vi "SDSU_SetInitVals.vi"(0 "ConfigPath":path, 11 "error in":errorcluster) -> (6 "supabort":bool, 8 "libdir out":path, 10 "cmdtrans out":path, 15 "error out":errorcluster)   [LabVIEW 2016]
uses:
  DHE/private/vis/DHE_Device.ctl
  SDSU_GBLVariables.vi
  DBSHAND/private/vis/DatabaseHand_Element_Set(string).vi
panel:
  in  "supinttime":bool
  in  "cmdtrans":path=path ""
  in  "devparams":string
  in  "libdir":path=path ""
  in  "linktype":string="genIII"
  in  "devtype":string="pcix"
  in  "mapsize":i32=-1
  in  "exp_overhead":string
  in  "minexptime":string
  in  "seq_overhead":string
  in  "Device In":T1 {"readtime" format="%.2f"}
  in  "suphardtime":bool
  in  "devno":i32
  in  "supabortctrl":bool
  in  "overhead":sgl=-1.0 format="%.2f"
  in  "ShiftedPix":i32=-1
  in  "bpp":i32=16
  in  "modifiers":string
  in  "FPA":string
  in  "readoutmode":string
  in  "ConfigVariables":string[][](table)=[["Device", "devno", "SDSU_SetInitVals.vi", "devno", "0", "I32"], ["Device", "mapsize", "SDSU_SetInitVals.vi", "mapsize", "", "I32"], ["Device", "params", "SDSU_SetInitVals.vi", "devparams", "", "STR"], ["Device", "type", "SDSU_SetInitVals.vi", "devtype", "", "STR"], ["Device", "link", "SDSU_SetInitVals.vi", "linktype", "", "STR"], ["Device", "libdir", "SDSU_SetInitVals.vi", "libdir", "", "Path"], ["Lod", "Utility", "SDSU_SetInitVals.vi", "Utility Path", "none", "Path"], ["Lod", "Timing", "SDSU_SetInitVals.vi", "Timing Path", "none", "Path"], ["Lod", "Pci", "SDSU_SetInitVals.vi", "Pci Path", "none", "Path"], ["Geometry", "FPA", "SDSU_SetInitVals.vi", "FPA", "", "STR"], ["Geometry", "modifiers", "SDSU_SetInitVals.vi", "modifiers", "", "STR"], ["FPA", "name", "SDSU_SetInitVals.vi", "FPA", "", "STR"], ["FPA", "modifiers", "SDSU_SetInitVals.vi", "modifiers", "", "STR"], ["FPA", "readmode", "SDSU_SetInitVals.vi", "readoutmode", "", "STR"], ["Roi", "Xstart", "SDSU_SetInitVals.vi", "xstart", "1", "U32"], ["Roi", "Xsize", "SDSU_SetInitVals.vi", "xsize", "2048", "U32"], ["Roi", "Ystart", "SDSU_SetInitVals.vi", "ystart", "1", "U32"], ["Roi", "Ysize", "SDSU_SetInitVals.vi", "ysize", "2048", "U32"], ["Binning", "X", "SDSU_SetInitVals.vi", "xbin", "1", "U32"], ["Binning", "Y", "SDSU_SetInitVals.vi", "ybin", "1", "U32"], ["Misc", "ReadoutMode", "SDSU_SetInitVals.vi", "readoutmode", "left", "STR"], ["Misc", "Temperature", "SDSU_SetInitVals.vi", "CCDTemperature", "-110", "I32"], ["Misc", "Commands", "SDSU_SetInitVals.vi", "CommandStr", "", "STR"], ["Misc", "bpp", "SDSU_SetInitVals.vi", "bpp", "16", "I32"], ["Misc", "min_exptime", "SDSU_SetInitVals.vi", "min_exptime", "0", "SGL"], ["Misc", "transfile", "SDSU_SetInitVals.vi", "cmdtrans", "", "PATH"], ["Readout", "PixelTime", "SDSU_SetInitVals.vi", "PixelTime", "3", "SGL"], ["Readout", "SkipPixel", "SDSU_SetInitVals.vi", "SkipPixel", "0", "SGL"], ["Readout", "SkipRow", "SDSU_SetInitVals.vi", "SkipRow", "0", "SGL"], ["Readout", "ShiftRow", "SDSU_SetInitVals.vi", "ShiftRow", "0", "SGL"], ["Readout", "ShiftedPix", "SDSU_SetInitVals.vi", "ShiftedPix", "0", "I32"], ["Readout", "known_overhead", "SDSU_SetInitVals.vi", "overhead", "0", "SGL"], ["Readout", "frame_overhead", "SDSU_SetInitVals.vi", "overhead", "0", "SGL"], ["Readout", "seq_overhead", "SDSU_SetInitVals.vi", "seq_overhead", "0", "STR"], ["Readout", "exp_overhead", "SDSU_SetInitVals.vi", "exp_overhead", "0", "STR"], ["Readout", "minexptime", "SDSU_SetInitVals.vi", "minexptime", "0", "STR"], ["Readout", "support_abort", "SDSU_SetInitVals.vi", "supabortctrl", "", "BOOL"], ["Readout", "support_hardtime", "SDSU_SetInitVals.vi", "suphardtime", "", "BOOL"], ["Readout", "support_actual_inttime", "SDSU_SetInitVals.vi", "supinttime", "", "BOOL"]]
  in  "Pci Path":path=path "none"
  in  "ShiftRow":sgl=-1.0 format="%.2f"
  in  "SkipRow":sgl=-1.0 format="%.2f"
  in  "SkipPixel":sgl=-1.0 format="%.2f"
  in  "PixelTime":sgl=-1.0 format="%.2f"
  in  "CommandStr":string
  in  "min_exptime":sgl
  in  "Commnds To Execute after set":i32(listbox)
  in  "Timing Path":path=path "none"
  in  "Utility Path":path=path "none"
  in  "CCDTemperature":i32=-110
  # "Misc"
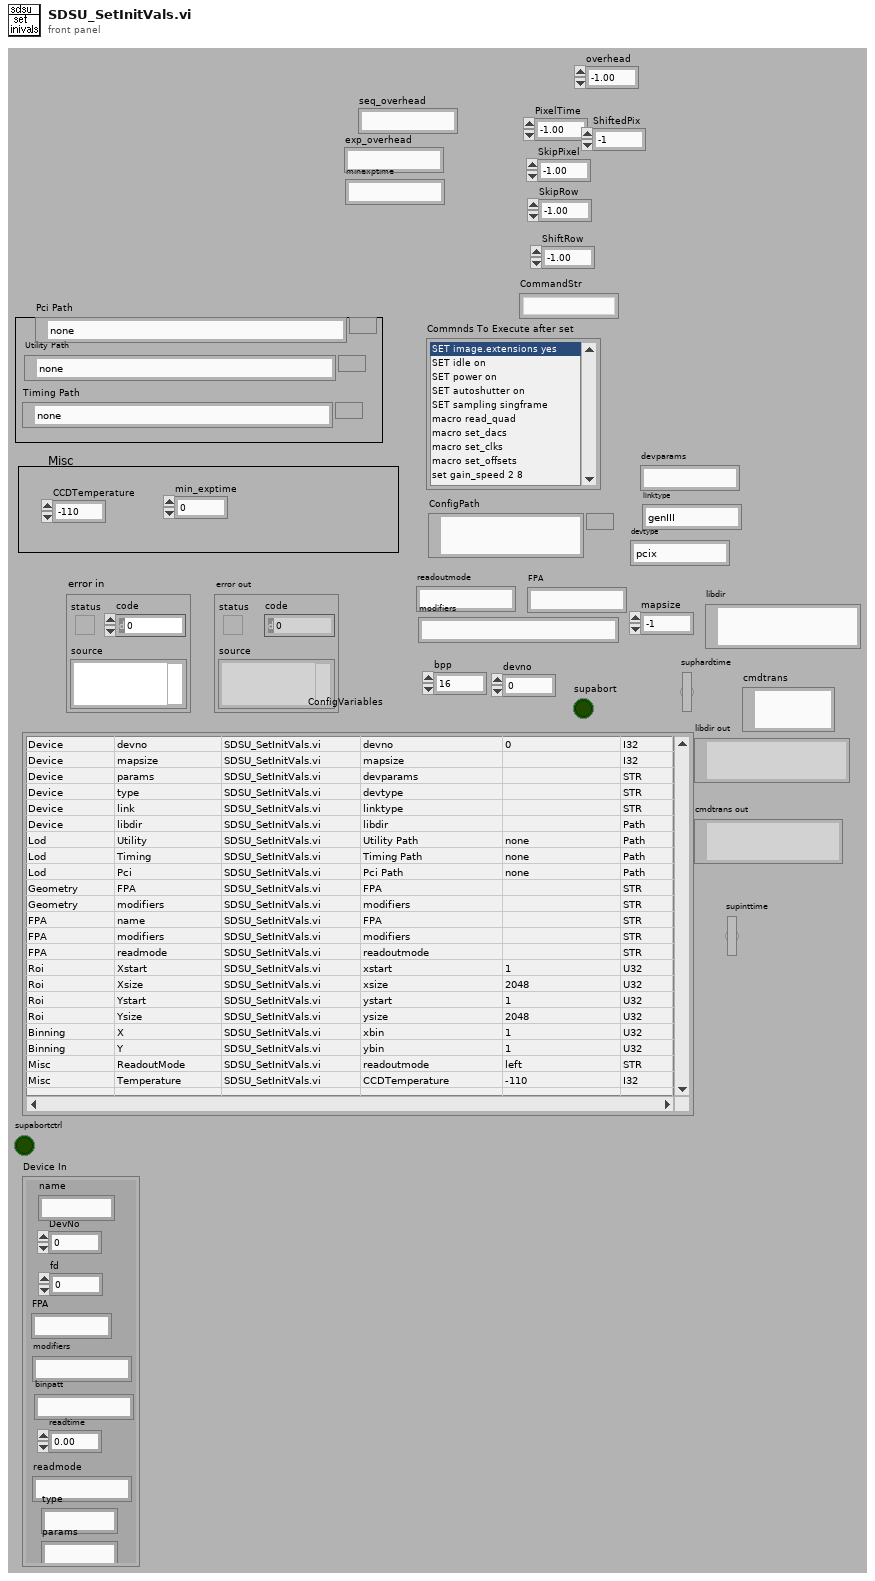
[diagram p1: front panel]
types:
  T1 = typedef "DHE_Device.ctl" = cluster{"DevNo":i32, "fd":i32, "name":string, "FPA":string, "modifiers":string, "binpatt":string, "readtime":dbl, "readmode":string, "type":string, "params":string}
  T2 = typedef "DatabaseHand_RefNum.ctl" = refnum<vi>
  T3 = enum16{"get fd", "set fd", "add ", "set_readtime", "get all", "clean all", "get by fd"}
  T4 = typedef "CMN_TimingInfo.ctl" = cluster{"PixelTime":sgl, "SkipPixel":sgl, "SkipRow":sgl, "ShiftRow":sgl, "ShiftedPix":u16, "known_overhead":sgl, "DET_READ_TIME":sgl}
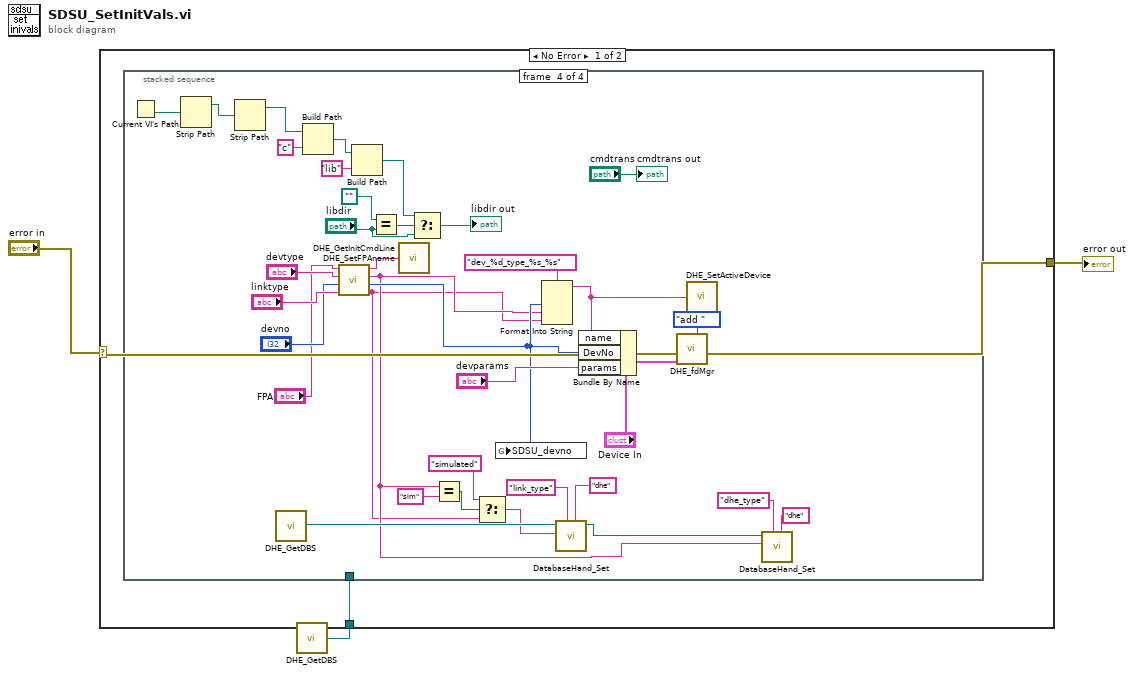
[diagram p0: block diagram]
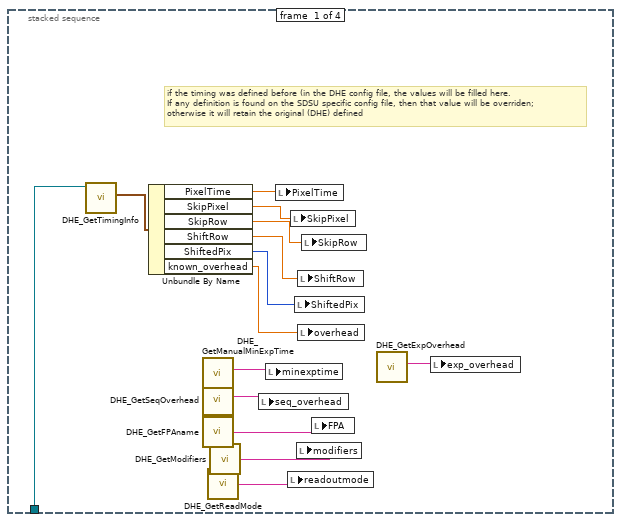
[diagram p2: hidden frame]
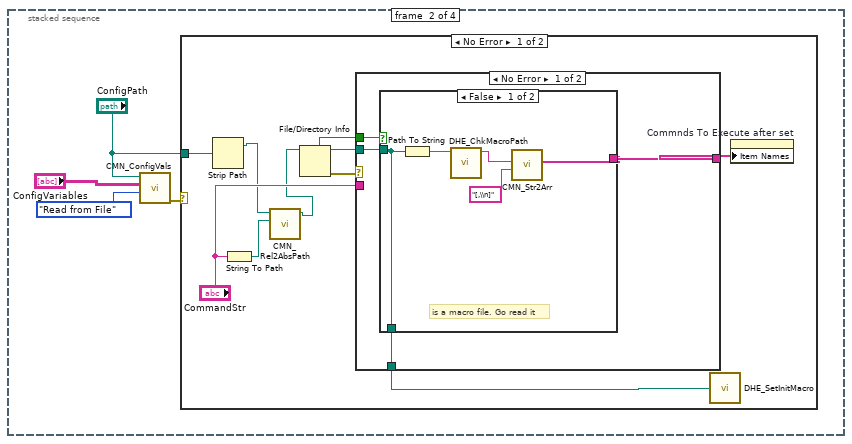
[diagram p3: hidden frame]
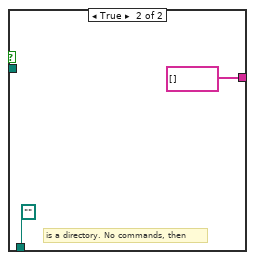
[diagram p4: hidden frame]
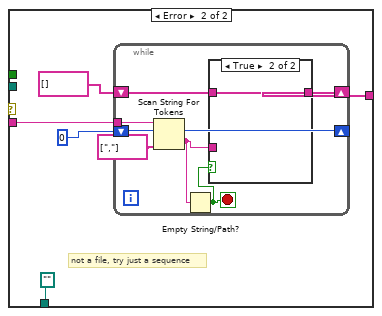
[diagram p5: hidden frame]
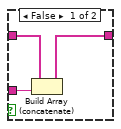
[diagram p6: hidden frame]
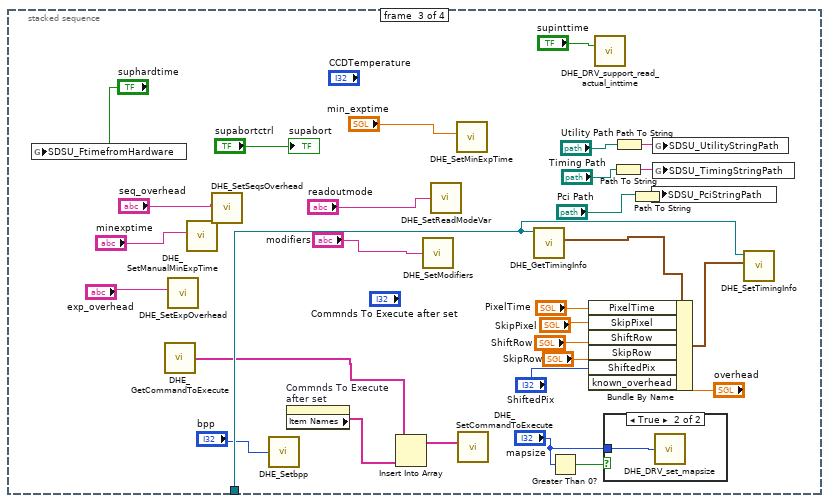
[diagram p8: hidden frame]
diagram:
  n1 = call "DHE_GetDBS.vi"() -> ("DHE_DBSRef"=w1:T2)  [unwired: 9 out]
  n2 = case shown="No Error" "error in" {
    selector: "error in" -> [w5 w129]
    tunnel: [w5 w129] -> w2
    tunnel: w1 -> [w4 _]
    frame No Error {
      n3 = stacked-sequence {
        tunnel: w4 -> [w19 _ w74 _]
        frame #0 {
          # "if the timing was defined before (in the DHE config file, the values will be filled here.\nIf any definition is found on the SDSU specific config file, then that value will be overriden;\notherwise it will retain the original (DHE) defined"
          n4 = call "DHE_GetTimingInfo.vi"("Database RefNum out"=w19) -> ("Timing"=w18:T4)  [unwired: 10 out]
          n5 = Unbundle By Name(w18) -> ("PixelTime"=w17:sgl, "SkipPixel"=w16:sgl, "SkipRow"=w15:sgl, "ShiftRow"=w14:sgl, "ShiftedPix"=w13:u16, "known_overhead"=w12:sgl)
          n6 = call "DHE_GetManualMinExpTime.vi"() -> ("ManualMinExpTime"=w10:string)  [unwired: 11 out]
          n7 = call "DHE_GetSeqOverhead.vi"() -> ("SeqOverhead"=w11:string)  [unwired: 11 out]
          n8 = call "DHE_GetFPAname.vi"() -> ("DHE_FPAname"=w7:string)  [unwired: 9 out]
          n9 = call "DHE_GetReadMode.vi"() -> ("DHE_ReadMode"=w9:string)  [unwired: 9 out]
          n10 = call "DHE_GetModifiers.vi"() -> ("DHE_Modifiers"=w8:string)  [unwired: 9 out]
          n11 = local write "seq_overhead"(w11) -> ()
          n12 = local write "minexptime"(w10) -> ()
          n13 = local write "PixelTime"(w17) -> ()
          n14 = local write "readoutmode"(w9) -> ()
          n15 = local write "SkipPixel"(w16) -> ()
          n16 = local write "ShiftedPix"(w13) -> ()
          n17 = local write "modifiers"(w8) -> ()
          n18 = local write "ShiftRow"(w14) -> ()
          n19 = local write "overhead"(w12) -> ()
          n20 = local write "SkipRow"(w15) -> ()
          n21 = local write "FPA"(w7) -> ()
          n22 = call "DHE_GetExpOverhead.vi"() -> ("ExpOverhead"=w6:string)  [unwired: 11 out]
          n23 = local write "exp_overhead"(w6) -> ()
        }
        frame #1 {
          n24 = call "CMN_ConfigVals.vi"("Action"=enum16{"Read from File", "Write to File"}."Read from File", "ConfigVariables"="ConfigVariables", "configuration file path"="ConfigPath") -> ("error out"=w23:errorcluster)  [unwired: 1 in, 7 out]
          n25 = case shown="No Error" w23 {
            tunnel: "ConfigPath" -> [w28 _]
            frame No Error {
              n26 = Strip Path(path=w28) -> (stripped path=w27:path)  [unwired: 1 out]
              n27 = String To Path(string="CommandStr") -> (path=w26:path)
              n28 = call "CMN_Rel2AbsPath.vi"("test path"=w26, "absolute path"=w27) -> ("output path"=w25:path)  [unwired: 1 in, 8 out]
              n29 = File/Directory Info(path=w25) -> (path out=w30:path, directory=w31:bool, error out=w32:errorcluster)  [unwired: 1 in, 4 out]
              n30 = case shown="No Error" w32 {
                tunnel: "CommandStr" -> [_ w49]
                tunnel: [w36 w46] -> w33
                tunnel: w31 -> [w37 _]
                tunnel: w30 -> [w35 _]
                tunnel: [w34 path ""] -> w24
                frame No Error {
                  n31 = case shown="False" w37 {
                    tunnel: [w42 string[] []] -> w36
                    tunnel: w35 -> [w40 _]
                    tunnel: [w40 path ""] -> w34
                    frame False {
                      # "is a macro file. Go read it"
                      n32 = Path To String(path=w40) -> (string=w39:string)
                      n33 = call "DHE_ChkMacroPath.vi"("macro name"=w39) -> ("macro out"=w38:string)  [unwired: 1 in, 9 out]
                      n34 = call "CMN_Str2Arr.vi"("separator"="[,\\n]", "string in"=w38) -> ("Array out"=w42:string[])  [unwired: 2 in, 7 out]
                    }
                    frame True {
                      # "is a directory. No commands, then"
                    }
                  }
                }
                frame Error {
                  # "not a file, try just a sequence"
                  n35 = while {
                    shift-left: 0 -> [w54]
                    shift-right: [w53] -> _
                    tunnel: w49 -> [w55]
                    shift-left: string[] [] -> [w51]
                    shift-right: [w57] -> w46
                    stop <- w50 stop-if-true
                    n36 = Scan String For Tokens(6:string[] [","] ("delimiters (\\s,\\t,\\r,\\n)"), 8:w54, 9:w55) -> (1:w52:string, 2:w53:i32)  [unwired: 5 out]
                    n37 = Empty String/Path?(string/path=w52) -> (empty?=w50:bool)
                    n38 = case shown="True" w50 {
                      tunnel: [w60 w61] -> w57
                      tunnel: w52 -> [w59 _]
                      tunnel: w51 -> [w58 w61]
                      frame False {
                        n39 = Build Array (concatenate)(w58, w59) -> (w60:string[])
                      }
                      frame True {
                      }
                    }
                  }
                }
              }
              n40 = call "DHE_SetInitMacro.vi"("DHE_InitMacro"=w24) -> ()  [unwired: 9 out]
              n41 = property on="Commnds To Execute after set" class="LstBox (strict)"("Item Names"=w33) -> ()  [unwired: 2 in, 2 out]
            }
            frame Error {
            }
          }
        }
        frame #2 {
          n42 = global write "SDSU_GBLVariables.vi" "SDSU_FtimefromHardware"("suphardtime") -> ()
          n43 = call "DHE_GetCommandToExecute.vi"() -> ("DHE_Commands2Exec"=w71:string[])  [unwired: 9 out]
          n44 = call "DHE_SetExpOverhead.vi"("ExpOverhead"="exp_overhead") -> ()  [unwired: 11 out]
          n45 = call "DHE_SetManualMinExpTime.vi"("ManualMinExptime"="minexptime") -> ()  [unwired: 11 out]
          n46 = call "DHE_SetSeqsOverhead.vi"("SeqsOverhead"="seq_overhead") -> ()  [unwired: 11 out]
          n47 = call "DHE_Setbpp.vi"("DHE_bpp"="bpp") -> ()  [unwired: 9 out]
          n48 = property on="Commnds To Execute after set" class="LstBox (strict)"() -> ("Item Names"=w81:string[])  [unwired: 2 in, 2 out]
          n49 = Insert Into Array(array=w71, new element=w81) -> (w70:string[])  [unwired: 1 in]
          n50 = call "DHE_SetModifiers.vi"("DHE_Modifiers"="modifiers") -> ()  [unwired: 9 out]
          n51 = call "DHE_SetReadModeVar.vi"("DHE_ReadMode"="readoutmode") -> ()  [unwired: 9 out]
          n52 = call "DHE_SetMinExpTime.vi"("MinExpTime"="min_exptime") -> ()  [unwired: 11 out]
          n53 = call "DHE_SetCommandToExecute.vi"("DHE_Commands2Exec"=w70) -> ()  [unwired: 9 out]
          n54 = call "DHE_GetTimingInfo.vi"("Database RefNum out"=w74) -> ("Timing"=w76:T4)  [unwired: 10 out]
          n55 = Greater Than 0?(x="mapsize") -> (x > 0?=w64:bool)
          n56 = Bundle By Name(cluster=w76, "PixelTime"="PixelTime", "SkipPixel"="SkipPixel", "ShiftRow"="ShiftRow", "SkipRow"="SkipRow", "ShiftedPix"="ShiftedPix", "known_overhead"="overhead") -> (w75:T4)
          n57 = call "DHE_DRV_support_read_actual_inttime.vi"("support rit?"="supinttime") -> ()  [unwired: 1 in, 14 out]
          n58 = case shown="True" w64 {
            tunnel: "mapsize" -> [_ w92]
            frame False {
            }
            frame True {
              n59 = call "DHE_DRV_set_mapsize.vi"("size_MB"=w92) -> ()  [unwired: 1 in, 14 out]
            }
          }
          n60 = Path To String(path="Timing Path") -> (string=w88:string)
          n61 = Path To String(path="Utility Path") -> (string=w91:string)
          n62 = Path To String(path="Pci Path") -> (string=w83:string)
          n63 = global write "SDSU_GBLVariables.vi" "SDSU_PciStringPath"(w83) -> ()
          n64 = global write "SDSU_GBLVariables.vi" "SDSU_UtilityStringPath"(w91) -> ()
          n65 = global write "SDSU_GBLVariables.vi" "SDSU_TimingStringPath"(w88) -> ()
          n66 = call "DHE_SetTimingInfo.vi"("Timing"=w75, "Database RefNum out"=w74) -> ()  [unwired: 10 out]
          "supabort" <- "supabortctrl"
        }
        frame #3 {
          n67 = Current VI's Path() -> (path=w119:path)
          n68 = Strip Path(path=w119) -> (stripped path=w118:path)  [unwired: 1 out]
          n69 = Strip Path(path=w118) -> (stripped path=w117:path)  [unwired: 1 out]
          n70 = call "DHE_GetDBS.vi"() -> ("DHE_DBSRef"=w104:T2)  [unwired: 9 out]
          n71 = Build Path(base path=w117, name or relative path="c") -> (appended path=w115:path)
          n72 = call "DHE_GetInitCmdLine.vi"("link"="linktype", "devno"="devno", "type"="devtype", "fpa in"="FPA") -> ("link out"=w95:string, "devno out"=w108:i32, "type out"=w98:string, "fpa out"=w106:string)  [unwired: 4 out]
          n73 = Build Path(base path=w115, name or relative path="lib") -> (appended path=w113:path)
          n74 = Equal?(x=path "", y="libdir") -> (x = y?=w128:bool)
          n75 = call "DHE_SetFPAname.vi"("DHE_FPAname"=w106) -> ()  [unwired: 1 in, 8 out]
          n76 = Select(t=w113, s=w128, f="libdir") -> (s? t:f=→"libdir out":path)
          n77 = Equal?(x=w98, y="sim") -> (x = y?=w96:bool)
          n78 = Select(t="simulated", s=w96, f=w95) -> (s? t:f=w94:string)
          n79 = global write "SDSU_GBLVariables.vi" "SDSU_devno"(w108) -> ()
          n80 = Format Into String(format string="dev_%d_type_%s_%s", w108, w98, w95) -> (resulting string=w123:string)  [unwired: 2 in, 1 out]
          n81 = call-poly "DatabaseHand_Set.vi"("group"="dhe", "name"="link_type", "value"=w94, "Database RefNum in"=w104) -> ("Database RefNum out"=w101:T2)  [unwired: 4 in, 3 out]
          n82 = Bundle By Name(cluster="Device In", "name"=w123, "DevNo"=w108, "params"="devparams") -> (w126:T1)
          n83 = call "DHE_fdMgr.vi"("Device In"=w126, "action"=T3."add ") -> ()  [unwired: 3 in, 7 out]
          n84 = call "DHE_SetActiveDevice.vi"("DHE_ActiveDevice"=w123) -> ()  [unwired: 9 out]
          n85 = call-poly "DatabaseHand_Set.vi"("group"="dhe", "name"="dhe_type", "value"=w98, "Database RefNum in"=w101) -> ()  [unwired: 4 in, 4 out]
          "cmdtrans out" <- "cmdtrans"
        }
      }
    }
    frame Error {
    }
  }
  "error out" <- w2
